vi "Find Workspace.vi"(8 "Error In":errorcluster, 10 "Control In":T2, 11 "Workspace In":refnum<class "Pick Up Tool Fixture.lvclass">) -> (0 "Error Out":errorcluster, 1 "Workspace Out":T1, 2 "Control Out":T2, 3 "Workspace Out":refnum<class "Pick Up Tool Fixture.lvclass">)   [LabVIEW 2019, in "Pick Up Tool Fixture.lvclass"]
uses:
  Pick Up Tool Fixture.lvclass
  C:/Users/HEP/Documents/Aerotech gantry/UCSB-Gantry-master/V5/Classes/Workspace/Fixture.lvclass
  Controller/Controllers.ctl
  Controller/I-O/I-O.lvclass
  Controller/Dispenser/Dispenser.lvclass
  C:/Program Files (x86)/Aerotech/A3200/LabVIEW/2010/Bin/Aerotech.A3200.dll
  Program Files (x86)/Aerotech/A3200/LabVIEW/2010/Bin/Aerotech.A3200.dll
  Workspace.ctl
  Fixture.lvclass/Fixture.ctl
  Read Position.vi
  Read Gantry Region.vi
  Fixture.lvclass
  Controller/Controller.lvclass
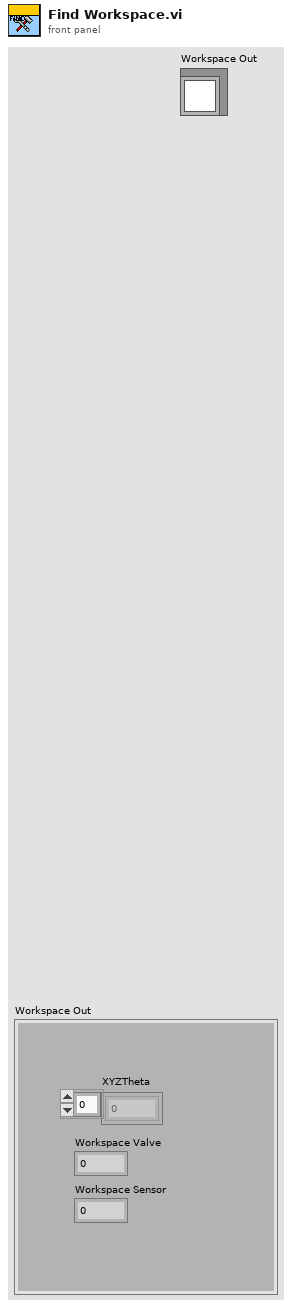
[diagram p1: front panel]
types:
  T1 = typedef "Fixture.lvclass/Workspace.ctl" = cluster{"XYZTheta":dbl[], "Workspace Valve":i32, "Workspace Sensor":i32}
  T2 = typedef "Controller.lvclass/Controllers.ctl" = cluster{"I-O.lvclass":refnum<class "I-O.lvclass">, "Dispenser.lvclass":refnum<class "Dispenser.lvclass">, "Gantry":refnum<k24>}
  T3 = typedef "File Paths.ctl" = cluster{"Glue Pattern Folder":path, "Carrier Tray Folder":path, "Pick Up Tool Fixture Folder":path, "Components Folder":path, "Bellows Tool Offset.txt":path, "Pick Up Tool Offset.txt":path, "Dispense Tip Offset.txt":path, "Log Files":path}
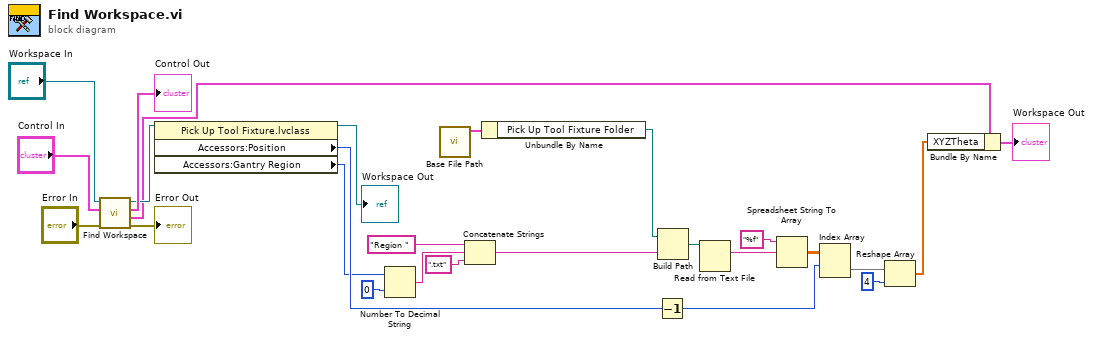
[diagram p0: block diagram]
diagram:
  n1 = call-parent "Find Workspace.vi"("Error In"="Error In", "Control In"="Control In", "Workspace In"="Workspace In") -> ("Error Out"=→"Error Out":errorcluster, 1:"Workspace Out"=w8:T1, "Control Out"=→"Control Out":T2, 3:"Workspace Out"=w20:refnum<class "Pick Up Tool Fixture.lvclass">)  [unwired: 5 in]
  n2 = property class="Pick Up Tool Fixture.lvclass"(reference=w20) -> (reference out=→"Workspace Out":refnum<class "Pick Up Tool Fixture.lvclass">, "Accessors:Position"=w4:i32, "Accessors:Gantry Region"=w2:i32)  [unwired: 1 in, 1 out]
  n3 = Number To Decimal String(number=w2, width (-)=i16 0) -> (decimal integer string=w18:string)
  n4 = call "Base File Path.vi"() -> ("Paths Out"=w21:T3)  [unwired: 11 in]
  n5 = Concatenate Strings("Region " ("string"), w18, ".txt") -> (w15:string)
  n6 = Unbundle By Name(w21) -> ("Pick Up Tool Fixture Folder"=w16:path)
  n7 = Decrement(x=w4) -> (x-1=w3:i32)
  n8 = Build Path(base path=w16, name or relative path=w15) -> (appended path=w14:path)
  n9 = Read from Text File(file (use dialog)=w14) -> (text=w13:string)  [unwired: 3 in, 3 out]
  n10 = Spreadsheet String To Array(format string="%f", spreadsheet string=w13) -> (array=w11:dbl[][])  [unwired: 2 in]
  n11 = Index Array(array=w11, index (row)=w3) -> (element=w10:dbl[])  [unwired: 1 in]
  n12 = Reshape Array(w10, 4 ("dimension size")) -> (w7:dbl[])
  n13 = Bundle By Name(cluster=w8, "XYZTheta"=w7) -> (→"Workspace Out":T1)
